vi "CRC-16（Input Hex String）.vi"(8 "error in (no error)":errorcluster caption="错误输入（无错误）", 11 "发送数据":string) -> (0 "error out":errorcluster caption="错误输出", 3 "完整命令":string)   [LabVIEW 2018]
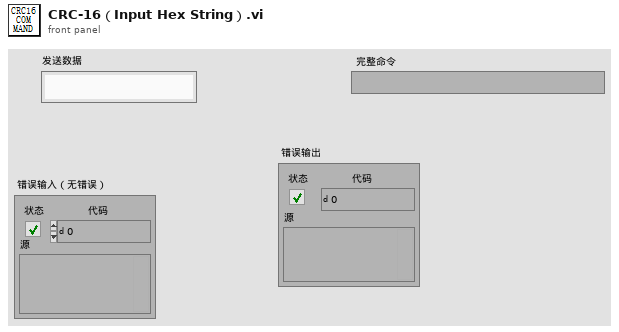
[diagram p1: front panel]
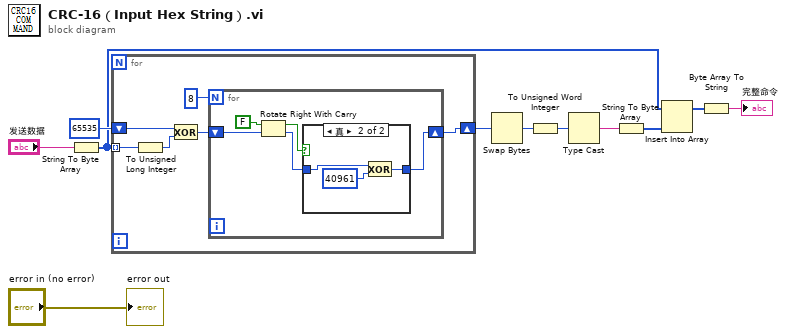
[diagram p0: block diagram]
diagram:
  n1 = String To Byte Array(string="发送数据") -> (unsigned byte array=w5:u8[])
  n2 = for {
    shift-right: [w14] -> w8
    shift-left: u32 65535 -> [w15]
    tunnel: w5 -> [w13] mode=indexing
    n3 = To Unsigned Long Integer(number=w13) -> (unsigned 32bit integer=w12:u32)
    n4 = Exclusive Or(1:w12, 2:w15) -> (0:w16:u32)
    n5 = for {
      N: 8 -> [_]
      shift-right: [w20] -> w14
      shift-left: w16 -> [w22]
      n6 = Rotate Right With Carry(2:w22, 3:FALSE) -> (0:w18:u32, 1:w19:bool)
      n7 = case shown="真" w19 {
        tunnel: w18 -> [w23 w25]
        tunnel: [w23 w24] -> w20
        frame False {
        }
        frame True {
          n8 = Exclusive Or(1:u32 40961, 2:w25) -> (0:w24:u32)
        }
      }
    }
  }
  n9 = Swap Bytes(anything=w8) -> (byte swapped=w6:u32)
  n10 = To Unsigned Word Integer(number=w6) -> (unsigned 16bit integer=w7:u16)
  n11 = Type Cast(x=w7) -> (*(type *) &x=w9:string)  [unwired: 1 in]
  n12 = String To Byte Array(string=w9) -> (unsigned byte array=w4:u8[])
  n13 = Insert Into Array(array=w5, new element=w4) -> (w3:u8[])  [unwired: 1 in]
  n14 = Byte Array To String(unsigned byte array=w3) -> (string=→"完整命令":string)
  "error out" <- "error in (no error)"
